vi "Set Owner.vi"(8 "error in (no error)":errorcluster, 10 "Owner":refnum<class>, 11 "ArrayPanel in":refnum<class "ArrayPanel.lvclass">) -> (0 "error out":errorcluster, 3 "ArrayPanel out":refnum<class "ArrayPanel.lvclass">)   [LabVIEW 2020, in "OOPanel.lvlib" / "ArrayPanel.lvclass"]
uses:
  ArrayPanel.lvclass
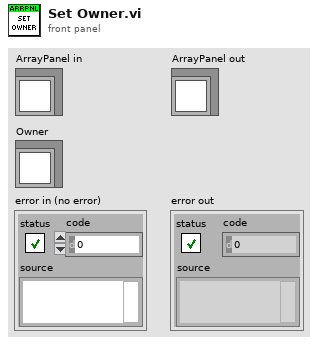
[diagram p1: front panel]
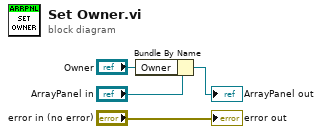
[diagram p0: block diagram]
diagram:
  n1 = Bundle By Name(cluster="ArrayPanel in", "Owner"="Owner") -> (→"ArrayPanel out":refnum<class "ArrayPanel.lvclass">)
  "error out" <- "error in (no error)"
